vi "Calculate S.vi"(8 "Frequency Bin (b)":dbl, 9 "Peak Frequencies":dbl[](array[numeric]), 10 "Peak Amplitudes":dbl[](array[numeric])) -> (2 "S":dbl)   [LabVIEW 2014]
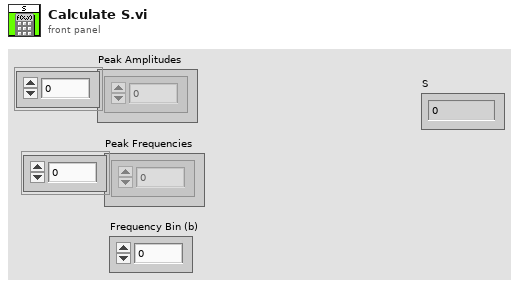
[diagram p1: front panel]
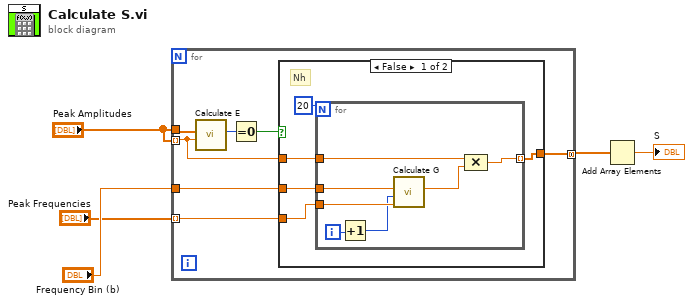
[diagram p0: block diagram]
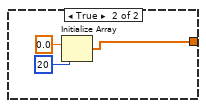
[diagram p2: hidden frame]
diagram:
  n1 = for {
    tunnel: "Peak Amplitudes" -> [w9]
    tunnel: "Frequency Bin (b)" -> [w12]
    tunnel: "Peak Amplitudes" -> [w6] mode=indexing
    tunnel: "Peak Frequencies" -> [w11] mode=indexing
    tunnel: [w10] -> w2 mode=concatenating
    n2 = call "Calculate E.vi"("Amplitude"=w6, "Peak Amplitudes"=w9) -> ("E"=w8:i32)  [unwired: 9 in]
    n3 = Equal To 0?(x=w8) -> (x = 0?=w7:bool)
    n4 = case shown="False" w7 {
      tunnel: w12 -> [w17 _]
      tunnel: w11 -> [w16 _]
      tunnel: [w14 w27] -> w10
      tunnel: w6 -> [w13 _]
      frame False {
        # "Nh"
        n5 = for {
          N: 20 -> [_]
          tunnel: w17 -> [w24]
          tunnel: w16 -> [w23]
          tunnel: [w19] -> w14 mode=indexing
          tunnel: w13 -> [w18]
          i -> [w21]
          n6 = Increment(x=w21) -> (x+1=w20:i32)
          n7 = call "Calculate G.vi"("Frequency (fihat)"=w23, "Subharmonic (h)"=w20, "Center frequency of bin (b)"=w24) -> ("G"=w22:dbl)  [unwired: 8 in]
          n8 = Compound Arithmetic op=MULTIPLY(w18, w22) -> (w19:dbl)
        }
      }
      frame True {
        n9 = Initialize Array(0.0 ("element"), 20 ("dimension size")) -> (w27:dbl[])
      }
    }
  }
  n10 = Add Array Elements(numeric array=w2) -> (sum=→"S":dbl)
